vi "Arm Stop.vi"(0 "Enum":enum16{"Init", "Run", "End"}(ring), 1 "Stop Arm":bool) -> ()   [LabVIEW 2011]
uses:
  TypeDefs/PWM Module 1.ctl
  <vilib>/Rock Robotics/SystemInterfaces/Typedef/FPGA_TypedefDigitalModule.ctl
  <vilib>/Rock Robotics/SystemInterfaces/DIO/FPGA_DIOPWMChannel.ctl
  <vilib>/Rock Robotics/SystemInterfaces/DIO/FPGA_DIORelayChannel.ctl
panel:
  in  "Angle":i32=105
  in  "PWM Module (DIO A)":T1={"Module"=enum."Digital Module 1", "Shooter Wheel"=enum."PWM 1", "Unassigned"=enum."PWM 2", "Unassigned"=enum."PWM 3", "Unassigned"=enum."PWM 4", "Unassigned"=enum."PWM 5", "Arm Servo"=enum."PWM 6", "Arm"=enum."PWM 7", "Ball Intake"=enum."PWM 8", "Conveyor Belt"=enum."PWM 9", "Shooter Feeder"=enum."PWM 10", "Camera Light"=enum."Relay 1", "Unassigned"=enum."Relay 2", "Unassigned"=enum."Relay 3", "Unassigned"=enum."Relay 4", "Unassigned"=enum."Relay 5", "Unassigned"=enum."Relay 6", "Unassigned"=enum."Relay 7", "Unassigned "=enum."Relay 8"}
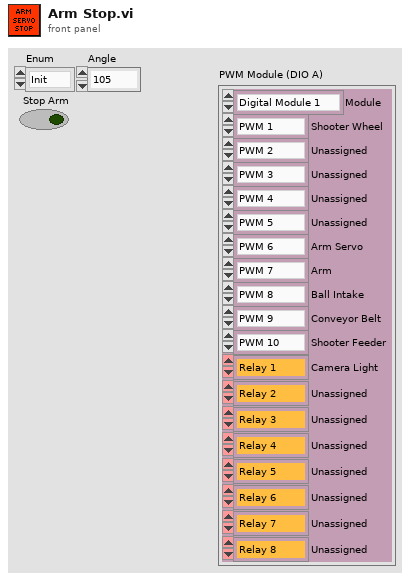
[diagram p1: front panel]
types:
  T1 = typedef "PWM Module 1.ctl" = cluster{"Module":T2, "Shooter Wheel":T3, "Unassigned":T3, "Unassigned":T3, "Unassigned":T3, "Unassigned":T3, "Arm Servo":T3, "Arm":T3, "Ball Intake":T3, "Conveyor Belt":T3, "Shooter Feeder":T3, "Camera Light":T4, "Unassigned":T4, "Unassigned":T4, "Unassigned":T4, "Unassigned":T4, "Unassigned":T4, "Unassigned":T4, "Unassigned ":T4}
  T2 = typedef "FPGA_TypedefDigitalModule.ctl" = enum16{"Digital Module 1", "Digital Module 2"}
  T3 = typedef "FPGA_DIOPWMChannel.ctl" = enum8{"PWM 1", "PWM 2", "PWM 3", "PWM 4", "PWM 5", "PWM 6", "PWM 7", "PWM 8", "PWM 9", "PWM 10", "Invalid"}
  T4 = typedef "FPGA_DIORelayChannel.ctl" = enum8{"Relay 1", "Relay 2", "Relay 3", "Relay 4", "Relay 5", "Relay 6", "Relay 7", "Relay 8", "Invalid"}
  T5 = typedef "WPI_ServoDeviceRef.ctl" = cluster{"DeviceStatus":errorcluster, "Digital Module":T2, "PWM Channel":T3, "DeadBand":T6}
  T6 = typedef "WPI_PWMDeadband.ctl" = cluster{"Name":string, "maxPositivePwm":i32, "minPositivePwm":i32, "centerPwm":i32, "maxNegativePwm":i32, "minNegativePwm":i32, "angularRange":u16}
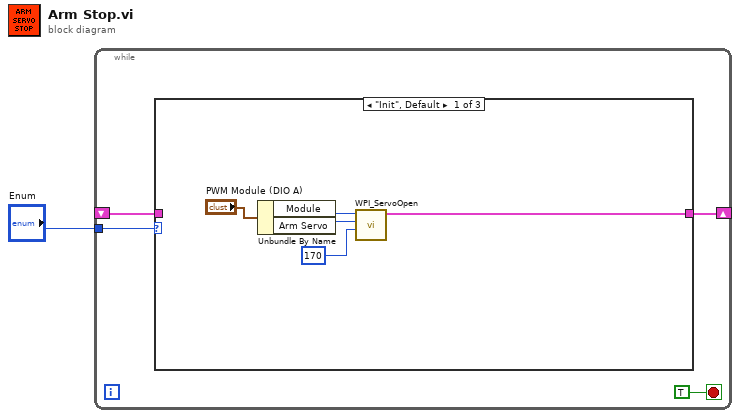
[diagram p0: block diagram]
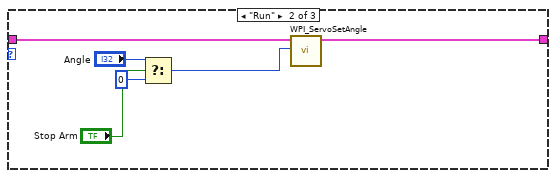
[diagram p2: hidden frame]
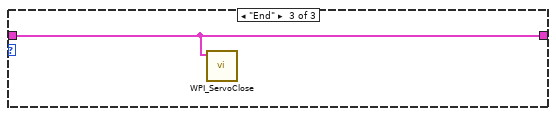
[diagram p3: hidden frame]
diagram:
  n1 = while {
    tunnel: "Enum" -> [w5]
    shift-right: [w4] -> _
    shift-left: _ -> [w3]
    stop <- TRUE stop-if-true
    n2 = case shown="\"Init\", Default" w5 {
      tunnel: [w6 w15 w17] -> w4
      tunnel: w3 -> [_ w16 w17]
      frame "Init", Default {
        n3 = Unbundle By Name("PWM Module (DIO A)") -> ("Module"=w9:T2, "Arm Servo"=w8:T3)
        n4 = call <vilib>:"WPI_ServoOpen.vi"("Angular Range"=u16 170, "PWM Channel"=w8, "Digital Module (Module 1)"=w9) -> ("ServoDeviceRef"=w6:T5)  [unwired: 7 in, 1 out]
      }
      frame "Run" {
        n5 = Select(t="Angle", s="Stop Arm", f=0) -> (s? t:f=w11:i32)
        n6 = call <vilib>:"WPI_ServoSetAngle.vi"("Angle"=w11, "ServoDeviceRef"=w16) -> ("ServoDeviceRef"=w15:T5)  [unwired: 8 in, 1 out]
      }
      frame "End" {
        n7 = call <vilib>:"WPI_ServoClose.vi"("MotorControlDevRef"=w17) -> ()  [unwired: 10 in, 1 out]
      }
    }
  }
